vi "Mod_OFDM_Complex Waveform_Generation.vi"(0 "Complex Symbols \nw/ Cyclic prefix":cdb[](array[numeric]), 5 "Parameters per Ofdm Symbol":T4 {"Data Source"."Data Source"."Register Initial State" format="%08x"}, 9 "Pulse Shaping":T3={"System Filter"={"TX Filter"=enum."Root Raised Cos", "Alpha"=0.5, "filter length"=8}, "Modulation system parameters"={"samples per symbol (16)"=16}, "symbol rate (Hz)"=1.0} {"symbol rate (Hz)" min=1.0 step=1.0 format="%.2p"; "Modulation system parameters"."samples per symbol (16)" step=2; "System Filter"."Alpha" min=0.0 max=1.0 step=0.05 format="%.2f"}, 11 "error in (no error)":errorcluster, 13 "Config_Waveform":T1={"Phase Continous \nWaveform"=FALSE, "Store Waveform\nTo a File"=FALSE, "Generate Waveform"=TRUE, "Store Waveform + \nConfiguration To Files"=FALSE}) -> (4 "output complex waveform":T2={"t0"=0.0, "dt"=1.0, "Y"=[]} {"Y" format="%.3f"; "dt" format="%^.2e"; "t0" format="%.4f"}, 6 "Parameters per Ofdm Symbol":T4 {"Data Source"."Data Source"."Register Initial State" format="%08x"}, 8 "matched filter coefficients":dbl[](array[numeric]) format="%.2f", 10 "Pulse Shaping":T3={"System Filter"={"TX Filter"=enum."Root Raised Cos", "Alpha"=0.5, "filter length"=8}, "Modulation system parameters"={"samples per symbol (16)"=16}, "symbol rate (Hz)"=1.0} {"symbol rate (Hz)" min=1.0 step=1.0 format="%.2p"; "Modulation system parameters"."samples per symbol (16)" step=2; "System Filter"."Alpha" min=0.0 max=1.0 step=0.05 format="%.2f"}, 15 "error out":errorcluster)   [LabVIEW 2010]
doc: "The VI applies pulse shaping based on the selected parameters for generating the complex waveform."
uses:
  Controls(Type_DEf)/Configure Pulse Shaping.ctl
  Controls(Type_DEf)/Parameters per Ofdm Symbol.ctl
  <vilib>/addons/Modulation/Analog/controls/Complex Data Waveform.ctl
  <vilib>/addons/Modulation/Digital/General/MT Apply Pulse Shaping Filter (Generic).vi
panel:
  in  "reset? (T)":bool=TRUE
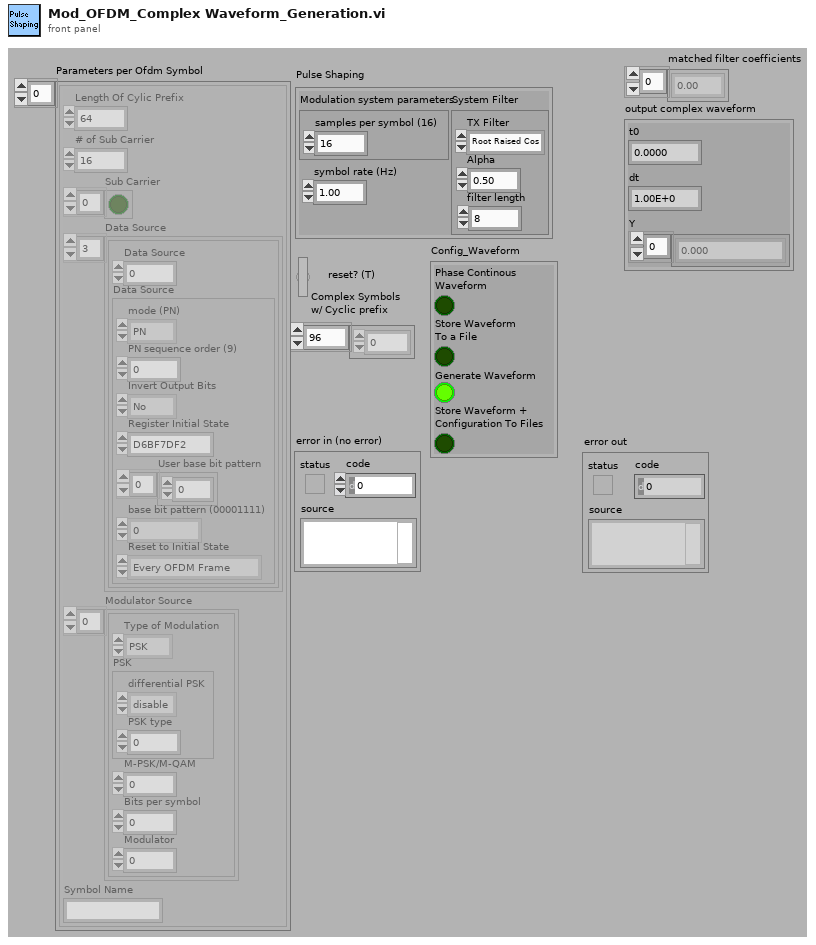
[diagram p1: front panel]
types:
  T1 = cluster{"Phase Continous \nWaveform":bool, "Store Waveform\nTo a File":bool, "Generate Waveform":bool, "Store Waveform + \nConfiguration To Files":bool}
  T2 = typedef "Complex Data Waveform.ctl" = cluster{"t0":dbl, "dt":dbl, "Y":cdb[]}
  T3 = typedef "Configure Pulse Shaping.ctl" = cluster{"System Filter":cluster{"TX Filter":enum16{"none", "Raised Cosine", "Root Raised Cos"}, "Alpha":dbl, "filter length":i32}, "Modulation system parameters":cluster{"samples per symbol (16)":u32}, "symbol rate (Hz)":dbl}
  T4 = typedef "Parameters per Ofdm Symbol.ctl" = cluster{"Length Of Cylic Prefix":i32, "# of Sub Carrier":i32, "Sub Carrier":bool[], "Data Source":cluster{"Data Source":u16, "Data Source":cluster{"mode (PN)":enum16{"PN", "pattern", "user"}, "PN sequence order (9)":i32, "Invert Output Bits":enum16{"No", "Yes"}, "Register Initial State":u32, "User base bit pattern":i8[], "base bit pattern (00001111)":enum16{"0", "1", "01", "0011", "00001111"}, "Reset to Initial State":enum16{"Every OFDM Frame", "Every OFDM Symbol", "Every Sub Carrier"}}}[], "Modulator Source":cluster{"Type of Modulation":enum16{"PSK", "QAM"}, "PSK":cluster{"differential PSK":enum16{"disable", "enable"}, "PSK type":u16}, "M-PSK/M-QAM":i32, "Bits per symbol":i32, "Modulator":u16}[], "Symbol Name":string}[]
  T5 = enum16{"none", "Raised Cosine", "Root Raised Cos"}
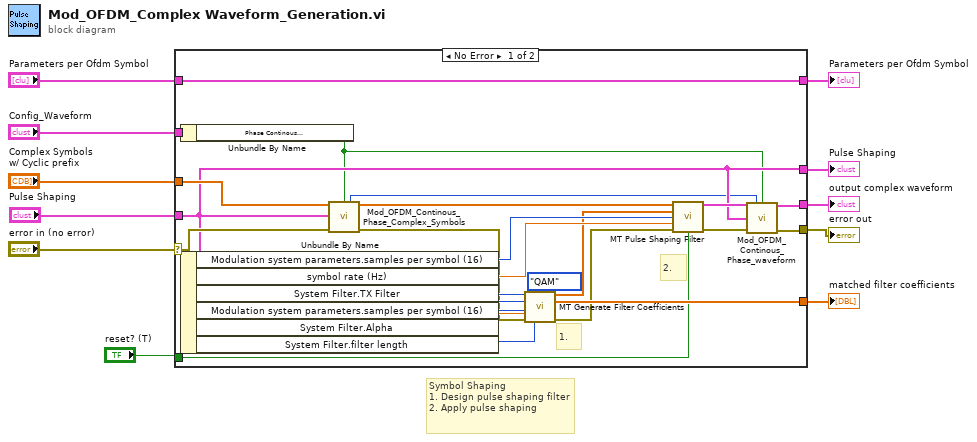
[diagram p0: block diagram]
diagram:
  # "Symbol Shaping\n1. Design pulse shaping filter\n2. Apply pulse shaping"
  n1 = case shown="No Error" "error in (no error)" {
    selector: "error in (no error)" -> [w23 w36]
    tunnel: "reset? (T)" -> [w29 _]
    tunnel: [w35 _] -> w10
    tunnel: [w16 w36] -> w1
    tunnel: "Pulse Shaping" -> [w15 _]
    tunnel: [w18 _] -> w4
    tunnel: [w33 _] -> w8
    tunnel: "Parameters per Ofdm Symbol" -> [w33 _]
    tunnel: [w15 _] -> w6
    tunnel: "Complex Symbols \nw/ Cyclic prefix" -> [w22 _]
    tunnel: "Config_Waveform" -> [w13 _]
    frame No Error {
      # "2."
      # "1."
      n2 = Unbundle By Name(w13) -> ("Phase Continous \nWaveform"=w12:bool)
      n3 = Unbundle By Name(w15) -> ("Modulation system parameters.samples per symbol (16)"=w31:u32, "symbol rate (Hz)"=w32:dbl, "System Filter.TX Filter"=w24:T5, "Modulation system parameters.samples per symbol (16)"=w25:u32, "System Filter.Alpha"=w26:dbl, "System Filter.filter length"=w27:i32)
      n4 = call "Mod_OFDM_Continous_Phase_Complex_Symbols.vi"("Complex Symbols w/ Cyclic prefix"=w22, "Phase Continous"=w12, "Pulse Shaping"=w15, "error in (no error)"=w23) -> ("Size of Complex Symbols"=w14:i32, "Complex Symbols w/ Cyclic prefix"=w20:cdb[], "error out"=w21:errorcluster)  [unwired: 9 in]
      n5 = call <vilib>:"MT Generate Filter Coefficients.vi"("pulse shaping filter (none)"=w24, "modulation type"=enum16{"FSK", "PSK", "QAM", "MSK", "PAM", "ASK"}."QAM", "pulse shaping samples per symbol (16)"=w25, "matched samples per symbol (16)"=w25, "filter parameter"=w26, "error in (no error)"=w21, "filter length (symbols)"=w27) -> ("pulse shaping filter coefficients"=w30:dbl[], "matched filter coefficients"=w35:dbl[], "error out"=w28:errorcluster)  [unwired: 6 in]
      n6 = call-poly <vilib>:"MT Pulse Shaping Filter.vi"("symbols"=w20, "pulse shaping filter coefficients"=w30, "samples per symbol (16)"=w31, "symbol rate (Hz)"=w32, "error in (no error)"=w28, "reset? (T)"=w29) -> ("output complex waveform"=w19:T2, "error out"=w17:errorcluster)  [unwired: 8 in]
      n7 = call "Mod_OFDM_Continous_Phase_waveform.vi"("Input Complex waveform"=w19, "Size of Complex Symbols"=w14, "Phase Continous"=w12, "Pulse Shaping"=w15, "error in (no error)"=w17) -> ("Complex waveform"=w18:T2, "error out"=w16:errorcluster)  [unwired: 9 in]
    }
    frame Error {
    }
  }
  "error out" <- w1
  "matched filter coefficients" <- w10
  "Parameters per Ofdm Symbol" <- w8
  "Pulse Shaping" <- w6
  "output complex waveform" <- w4
